vi "MD5Checksum core.vi"(7 "Input String":string, 8 "s4 in":u32=271733878 format="%.0x", 9 "s3 in":u32=2562383102 format="%.0x", 10 "s2 in":u32=4023233417 format="%.0x", 11 "s1 in":u32=1732584193 format="%.0x") -> (0 "s4 out":u32, 1 "s3 out":u32, 2 "s2 out":u32, 3 "s1 out":u32)   [LabVIEW 2016]
doc: "This VI contains the core of the MD5 algorithm."
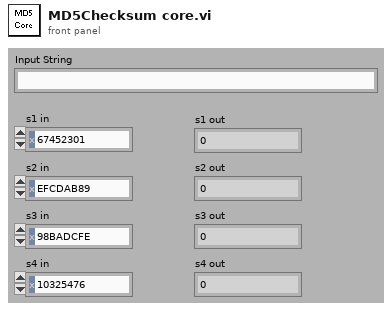
[diagram p1: front panel]
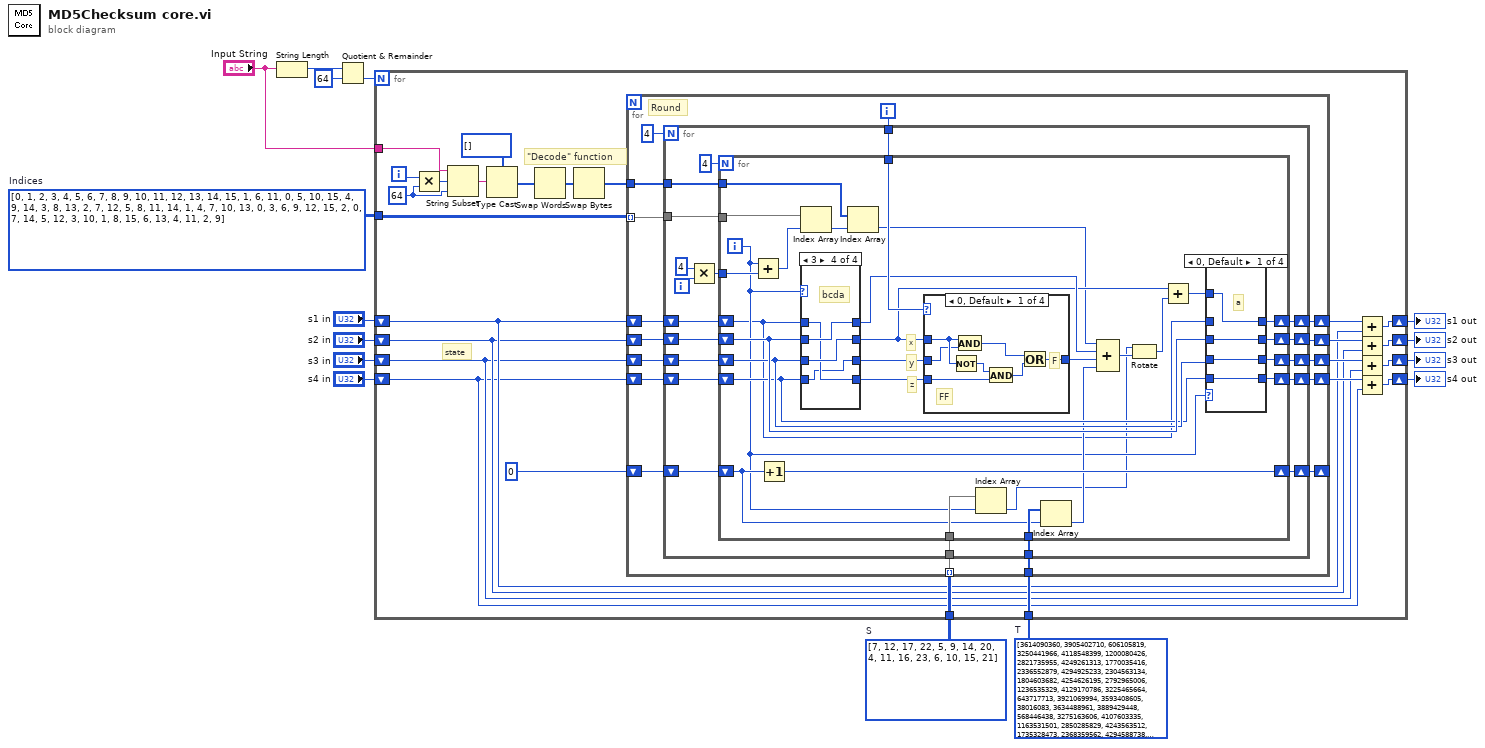
[diagram p0: block diagram]
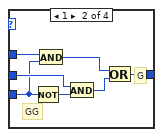
[diagram p2: hidden frame]
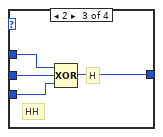
[diagram p3: hidden frame]
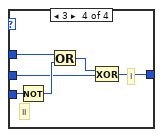
[diagram p4: hidden frame]
diagram:
  w9 = i32[][] [[7, 12, 17, 22], [5, 9, 14, 20], [4, 11, 16, 23], [6, 10, 15, 21]]  # S
  w10 = u32[] [3614090360, 3905402710, 606105819, 3250441966, 4118548399, 1200080426, 2821735955, 4249261313, 1770035416, 2336552879, 4294925233, 2304563134, 1804603682, 4254626195, 2792965006, 1236535329, 4129170786, 3225465664, 643717713, 3921069994, 3593408605, 38016083, 3634488961, 3889429448, 568446438, 3275163606, 4107603335, 1163531501, 2850285829, 4243563512, 1735328473, 2368359562, 4294588738, 2272392833, 1839030562, 4259657740, 2763975236, 1272893353, 4139469664, 3200236656, 681279174, 3936430074, 3572445317, 76029189, 3654602809, 3873151461, 530742520, 3299628645, 4096336452, 1126891415, 2878612391, 4237533241, 1700485571, 2399980690, 4293915773, 2240044497, 1873313359, 4264355552, 2734768916, 1309151649, 4149444226, 3174756917, 718787259, 3951481745]  # T
  w11 = i32[][] [[0, 1, 2, 3, 4, 5, 6, 7, 8, 9, 10, 11, 12, 13, 14, 15], [1, 6, 11, 0, 5, 10, 15, 4, 9, 14, 3, 8, 13, 2, 7, 12], [5, 8, 11, 14, 1, 4, 7, 10, 13, 0, 3, 6, 9, 12, 15, 2], [0, 7, 14, 5, 12, 3, 10, 1, 8, 15, 6, 13, 4, 11, 2, 9]]  # Indices
  n1 = String Length(string="Input String") -> (length=w14:i32)
  n2 = Quotient & Remainder(x=w14, y=64) -> (floor(x/y)=w15:i32)  [unwired: 1 out]
  n3 = for {
    N: w15 -> [_]
    tunnel: w11 -> [w35]
    tunnel: w10 -> [w34]
    tunnel: w9 -> [w33]
    shift-right: [w32] -> w8
    shift-left: "s1 in" -> [w28]
    shift-right: [w31] -> w7
    shift-left: "s2 in" -> [w27]
    shift-right: [w30] -> w6
    shift-left: "s3 in" -> [w26]
    shift-right: [w29] -> w5
    shift-left: "s4 in" -> [w25]
    tunnel: "Input String" -> [w23]
    i -> [w24]
    w19 = 64 ("y")
    # "\"Decode\" function"
    # "state"
    n4 = Multiply(x=w24, y=w19) -> (x*y=w20:i32)
    n5 = String Subset(string=w23, offset (0)=w20, length (rest)=w19) -> (substring=w22:string)
    n6 = Type Cast(type=u32[] [], x=w22) -> (*(type *) &x=w17:u32[])
    n7 = Swap Words(1:w17) -> (0:w18:u32[])
    n8 = Swap Bytes(anything=w18) -> (byte swapped=w16:u32[])
    n9 = for {
      shift-right: [w51] -> w37
      shift-left: w28 -> [w52]
      shift-right: [w50] -> w38
      shift-left: w27 -> [w53]
      shift-right: [w49] -> w39
      shift-left: w26 -> [w54]
      shift-right: [w48] -> w40
      shift-left: w25 -> [w55]
      tunnel: w35 -> [w47] mode=indexing
      tunnel: w33 -> [w46] mode=indexing
      tunnel: w16 -> [w45]
      shift-right: [w42] -> _
      shift-left: 0 -> [w43]
      tunnel: w34 -> [w41]
      i -> [w56]
      # "Round"
      n10 = for {
        N: 4 -> [_]
        tunnel: w56 -> [w75]
        shift-right: [w68] -> w48
        shift-left: w55 -> [w69]
        shift-right: [w67] -> w49
        shift-left: w54 -> [w70]
        shift-right: [w73] -> w50
        shift-left: w53 -> [w71]
        shift-right: [w74] -> w51
        shift-left: w52 -> [w72]
        tunnel: w47 -> [w66]
        tunnel: w46 -> [w65]
        tunnel: w45 -> [w61]
        shift-right: [w58] -> w42
        shift-left: w43 -> [w59]
        tunnel: w41 -> [w57]
        i -> [w64]
        n11 = Multiply(x=4, y=w64) -> (x*y=w62:i32)
        n12 = for {
          N: 4 -> [_]
          tunnel: w75 -> [w87]
          shift-right: [w97] -> w68
          shift-left: w69 -> [w92]
          shift-right: [w96] -> w67
          shift-left: w70 -> [w93]
          shift-right: [w95] -> w73
          shift-left: w71 -> [w94]
          shift-right: [w98] -> w74
          shift-left: w72 -> [w78]
          tunnel: w66 -> [w105]
          tunnel: w65 -> [w104]
          tunnel: w62 -> [w91]
          tunnel: w61 -> [w101]
          shift-right: [w88] -> w58
          shift-left: w59 -> [w89]
          tunnel: w57 -> [w90]
          i -> [w79]
          # "z"
          # "y"
          # "x"
          n13 = Add(x=w79, y=w91) -> (x+y=w103:i32)
          n14 = Increment(x=w89) -> (x+1=w88:i32)
          n15 = Index Array(array=w105, index=w103) -> (element=w102:i32)
          n16 = case shown="3" w79 {
            tunnel: w78 -> [w149 w152 w155 w159]
            tunnel: w94 -> [w148 w151 w154 w161]
            tunnel: w93 -> [w147 w150 w157 w160]
            tunnel: w92 -> [w146 w153 w156 w158]
            tunnel: [w149 w153 w157 w161] -> w82
            tunnel: [w148 w152 w156 w160] -> w81
            tunnel: [w147 w151 w155 w158] -> w100
            tunnel: [w146 w150 w154 w159] -> w99
            frame 0, Default {
              # "abcd"
            }
            frame 1 {
              # "dabc"
            }
            frame 2 {
              # "cdab"
            }
            frame 3 {
              # "bcda"
            }
          }
          n17 = Index Array(array=w101, index=w102) -> (element=w76:u32)
          n18 = case shown="0, Default" w87 {
            tunnel: w81 -> [w109 w115 w122 w126]
            tunnel: w100 -> [w108 w114 w123 w125]
            tunnel: w99 -> [w107 w113 w121 w124]
            tunnel: [w106 w116 w120 w127] -> w83
            frame 0, Default {
              # "FF"
              # "F"
              n19 = Not(x=w109) -> (.not. x?=w112:u32)
              n20 = And(x=w109, y=w108) -> (x .and. y?=w111:u32)
              n21 = And(x=w112, y=w107) -> (x .and. y?=w110:u32)
              n22 = Or(x=w111, y=w110) -> (x .or. y?=w106:u32)
            }
            frame 1 {
              # "GG"
              # "G"
              n23 = Not(x=w113) -> (.not. x?=w117:u32)
              n24 = And(x=w115, y=w113) -> (x .and. y?=w118:u32)
              n25 = And(x=w114, y=w117) -> (x .and. y?=w119:u32)
              n26 = Or(x=w118, y=w119) -> (x .or. y?=w116:u32)
            }
            frame 2 {
              # "H"
              # "HH"
              n27 = Compound Arithmetic op=XOR(w122, w123, w121) -> (w120:u32)
            }
            frame 3 {
              # "I"
              # "II"
              n28 = Not(x=w124) -> (.not. x?=w129:u32)
              n29 = Or(x=w126, y=w129) -> (x .or. y?=w128:u32)
              n30 = Exclusive Or(1:w125, 2:w128) -> (0:w127:u32)
            }
          }
          n31 = Index Array(array=w104, index=w79) -> (element=w77:i32)
          n32 = Index Array(array=w90, index=w89) -> (element=w84:u32)
          n33 = Compound Arithmetic op=ADD(w76, w82, w83, w84) -> (w86:u32)
          n34 = Rotate(1:w86, 2:w77) -> (0:w80:u32)
          n35 = Add(x=w81, y=w80) -> (x+y=w85:u32)
          n36 = case shown="0, Default" w79 {
            tunnel: w85 -> [w133 w137 w141 w145]
            tunnel: [w133 w136 w140 w144] -> w98
            tunnel: [w130 w137 w138 w142] -> w97
            tunnel: [w131 w134 w141 w143] -> w96
            tunnel: [w132 w135 w139 w145] -> w95
            tunnel: w78 -> [_ w136 w140 w144]
            tunnel: w94 -> [w132 w135 w139 _]
            tunnel: w93 -> [w131 w134 _ w143]
            tunnel: w92 -> [w130 _ w138 w142]
            frame 0, Default {
              # "a"
            }
            frame 1 {
              # "d"
            }
            frame 2 {
              # "c"
            }
            frame 3 {
              # "b"
            }
          }
        }
      }
    }
    n37 = Add(x=w37, y=w28) -> (x+y=w32:u32)
    n38 = Add(x=w38, y=w27) -> (x+y=w31:u32)
    n39 = Add(x=w39, y=w26) -> (x+y=w30:u32)
    n40 = Add(x=w40, y=w25) -> (x+y=w29:u32)
  }
  "s1 out" <- w8
  "s2 out" <- w7
  "s3 out" <- w6
  "s4 out" <- w5
